vi "set_subpattern.vi"(6 "diameter":dbl, 7 "height":dbl, 8 "error in (no error)":errorcluster, 9 "number of iteration points":dbl, 10 "winding number":dbl, 11 "FPGAWrapperMH120124RAPS_PXI7813R in":refnum<class "FPGAWrapperMH120124RAPS_PXI7813R.lvclass">) -> (0 "error out":errorcluster, 3 "FPGAWrapperMH120124RAPS_PXI7813R out":refnum<class "FPGAWrapperMH120124RAPS_PXI7813R.lvclass">)   [LabVIEW 2010, in "FPGAWrapperMH120124RAPS_PXI7813R.lvclass"]
uses:
  FPGAWrapperMH120124RAPS_PXI7813R.lvclass
  fpgaVIsAndControls/ellipsoid_parameters_cluster.ctl
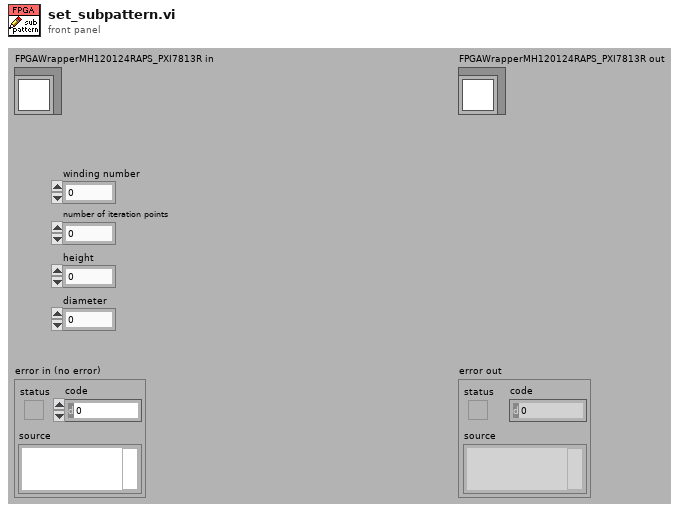
[diagram p1: front panel]
types:
  T1 = typedef "ellipsoid_parameters_cluster.ctl" = cluster{"a":fxp<+/-,16,1>, "b":fxp<+/-,16,1>, "c":fxp<+/-,16,1>, "d":fxp<+/-,16,1>, "e":fxp<+/-,24,16>, "k":u16, "width":fxp<+,16,16>}
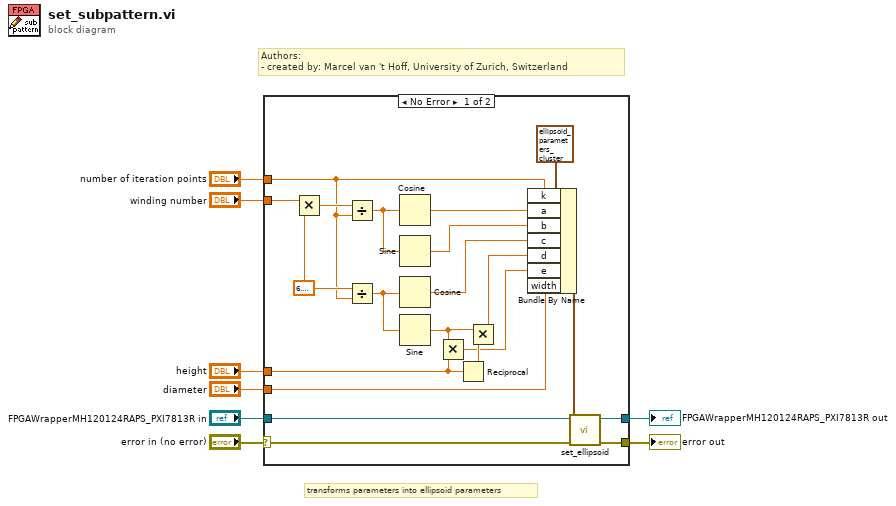
[diagram p0: block diagram]
diagram:
  # "transforms parameters into ellipsoid parameters"
  # "Authors: \n- created by: Marcel van 't Hoff, University of Zurich, Switzerland"
  n1 = case shown="No Error" "error in (no error)" {
    selector: "error in (no error)" -> [w27 w31]
    tunnel: [w26 w31] -> w7
    tunnel: [w28 w30] -> w5
    tunnel: "FPGAWrapperMH120124RAPS_PXI7813R in" -> [w29 w30]
    tunnel: "number of iteration points" -> [w9 _]
    tunnel: "winding number" -> [w23 _]
    tunnel: "height" -> [w12 _]
    tunnel: "diameter" -> [w10 _]
    frame No Error {
      w18 = 6.283185307179586
      n2 = Multiply(x=w23, y=w18) -> (x*y=w22:dbl)
      n3 = Divide(x=w22, y=w9) -> (x/y=w20:dbl)
      n4 = Divide(x=w18, y=w9) -> (x/y=w17:dbl)
      n5 = Cosine(x=w20) -> (cos(x)=w21:dbl)
      n6 = Sine(x=w20) -> (sin(x)=w19:dbl)
      n7 = Cosine(x=w17) -> (cos(x)=w16:dbl)
      n8 = Sine(x=w17) -> (sin(x)=w13:dbl)
      n9 = Multiply(x=w13, y=w12) -> (x*y=w11:dbl)
      n10 = Reciprocal(x=w12) -> (1/x=w15:dbl)
      n11 = Multiply(x=w13, y=w15) -> (x*y=w14:dbl)
      n12 = Bundle By Name(cluster=T1 {"a"=0.0, "b"=0.125, "c"=0.5, "d"=0.015625, "e"=0.5, "k"=0, "width"=0.0} ("ellipsoid parameter cluster"), "k"=w9, "a"=w21, "b"=w19, "c"=w16, "d"=w14, "e"=w11, "width"=w10) -> (w24:T1)
      n13 = call-dynamic "set_ellipsoid.vi"("error in (no error)"=w27, "ellipsoid parameter cluster"=w24, "FPGAWrapperMH120124RAPS_PXI7813R in"=w29) -> ("error out"=w26:errorcluster, "FPGAWrapperMH120124RAPS_PXI7813R out"=w28:refnum<class "FPGAWrapperMH120124RAPS_PXI7813R.lvclass">)  [unwired: 7 in]
    }
    frame Error {
    }
  }
  "error out" <- w7
  "FPGAWrapperMH120124RAPS_PXI7813R out" <- w5
